vi "Read Base Actor.vi"(11 "Actor in":refnum<class "Actor.lvclass">) -> (2 "Base Actor":refnum<data-value>)   [LabVIEW 2020, in "jettl.lvlib" / "Actor.lvclass"]
uses:
  Actor.lvclass
  Lifetime.ctl
  jettl.lvlib
  Base Actor.ctl
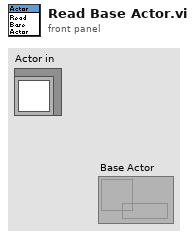
[diagram p1: front panel]
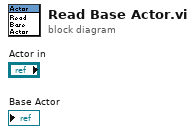
[diagram p0: block diagram]
diagram:
